vi "Main.vi"() -> ()   [LabVIEW 2023]
doc: "This template is for the Queued Message Handler design pattern.\n\nThe Event Handling Loop generates messages based on user interface actions.\n\nThe Message Handling Loop processes messages generated by the Event Handling Loop, or by other messages. The messages are string values, so new messages can be added easily to the Message Cases case structure in the Message Handling Loop. Each message cluster can also provide an optional value for Message Data, which is a variant that can be converted to whatever message-specific data is required."
uses:
  controls/UI Data.ctl
  support/Message Queue/Enqueue Message (Single).vi
  <vilib>/Utility/file.llb/Write Delimited Spreadsheet (string).vi
  <vilib>/Utility/file.llb/Write Delimited Spreadsheet (DBL).vi
  <vilib>/Instr/_visa.llb/VISA Configure Serial Port (Instr).vi
  <vilib>/Utility/error.llb/Error Cluster From Error Code.vi
  <vilib>/ErrorRing/Error Ring.xnode
  support/Message Queue/Message Queue.lvlib
  support/User Event - Stop/User Event - Stop.lvlib
panel:
  out "Acquiring Read":string
  in  "Step Time (ms)":dbl
  in  "Next Button":bool
  in  "Previous Button":bool
  in  "Test Case":string(combo)="standard"
  in  "File Path":path
  in  "Test Name":string
  out "Torque vs Displacement":cluster{dbl[], dbl[]}(graph)
  in  "COM Port":refnum<visa-resource-name>
  in  "Cycles":dbl
  in  "Torque":dbl
  in  "Microsteps":dbl
  in  "RPM":dbl
  in  "Clear":bool
  in  "Save":bool
  out "Status":string
  in  "Stop":bool
  in  "Start":bool
  in  "Exit":bool
  # "Settings"
  # "Test Controls"
  # "Manual Control"
  # "Torque vs Displacement"
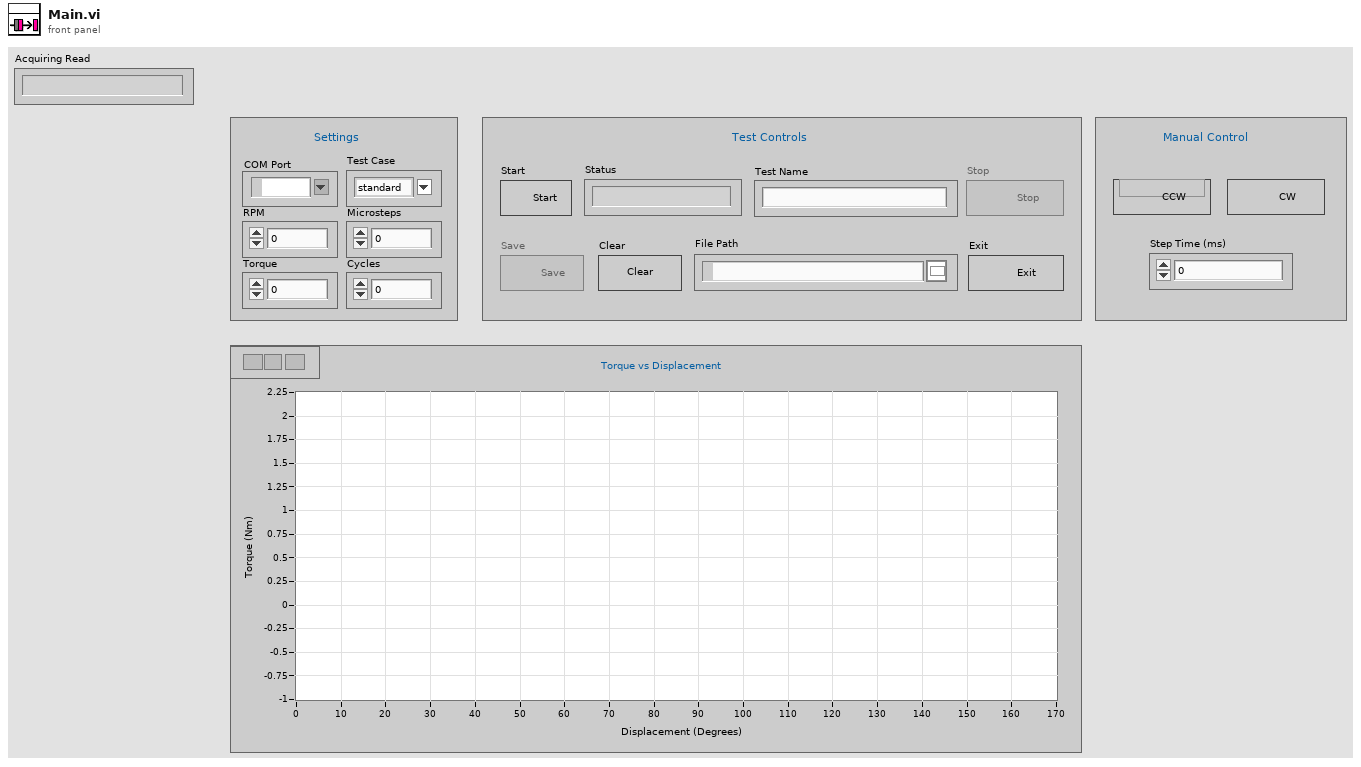
[diagram p1: front panel]
types:
  T1 = cluster{"RPM":dbl, "Microsteps":dbl, "Torque":dbl, "Cycles":dbl, "VISA resource name":refnum<visa-resource-name>, "test case":string}
  T2 = typedef "UI Data.ctl" = cluster{"Start ref":refnum<vi>, "Stop ref":refnum<vi>, "Status ref":refnum<vi>, "Exit ref":refnum<vi>, "Save ref":refnum<vi>, "Clear ref":refnum<vi>, "CCW":refnum<vi>, "CW":refnum<vi>}
  T3 = typedef "Message Queue.lvlib/All Message Queues.ctl" = cluster{"UI":refnum<queue>, "Acquisition":refnum<queue>}
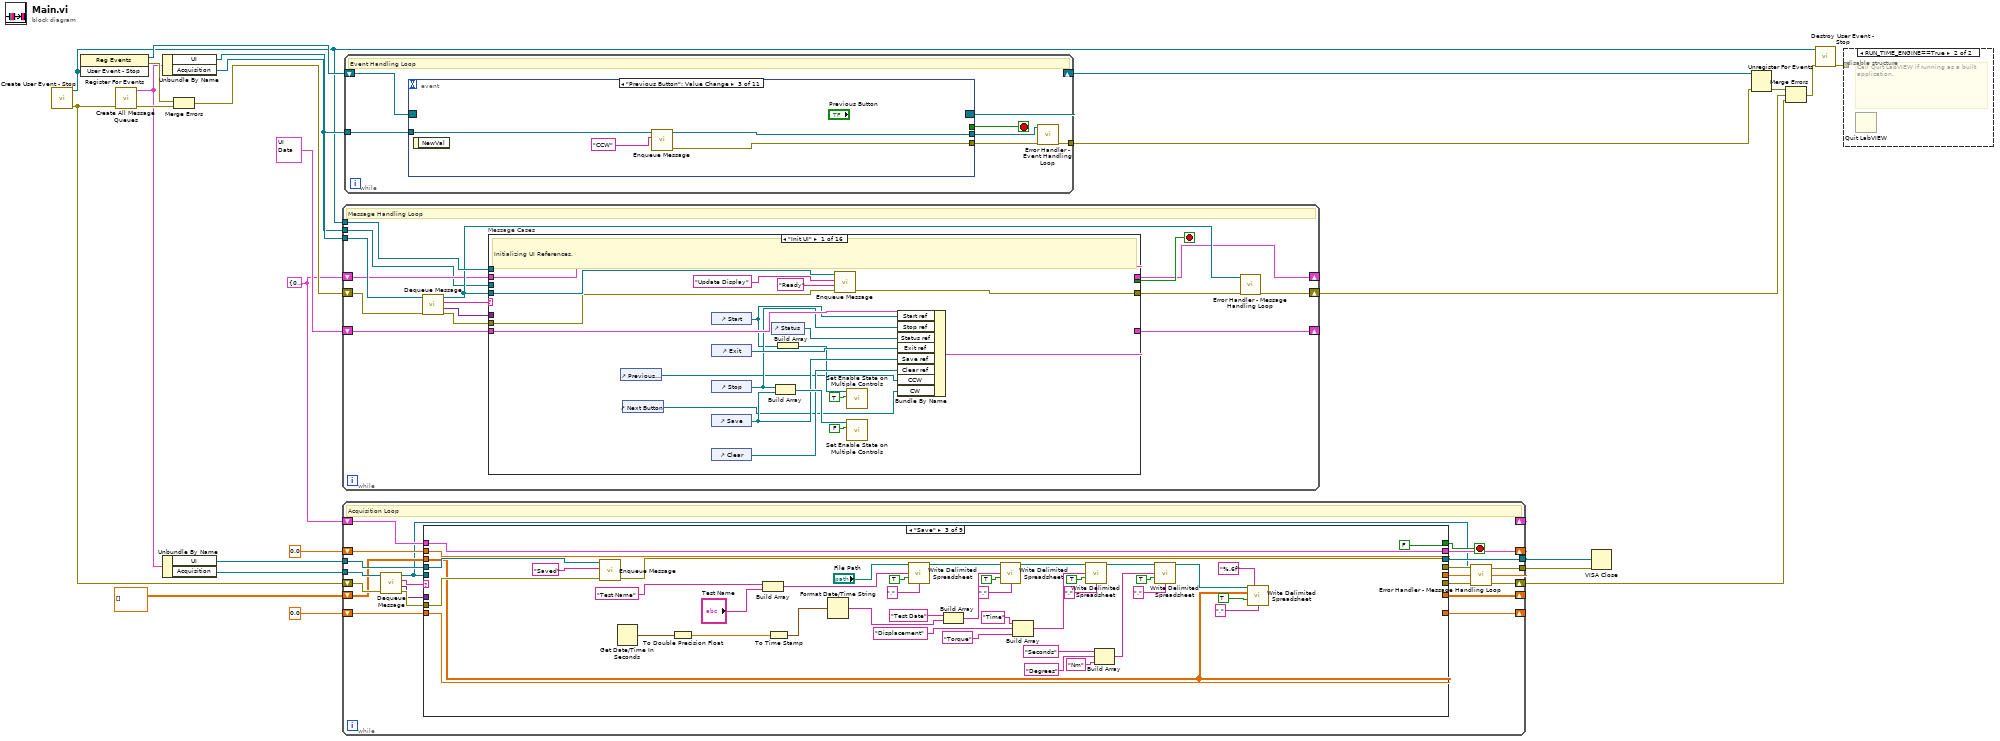
[diagram p0: block diagram]
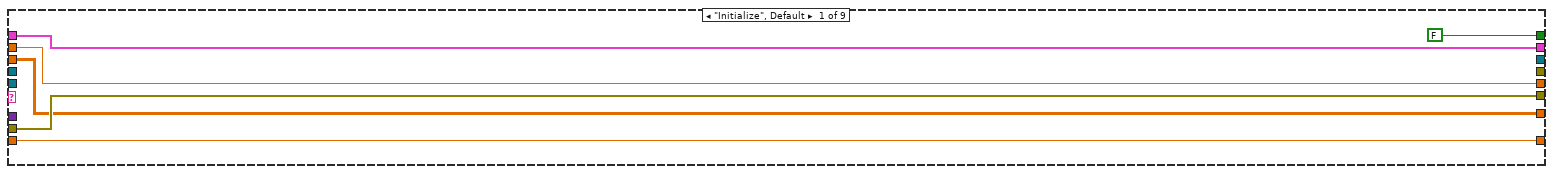
[diagram p2: hidden frame]
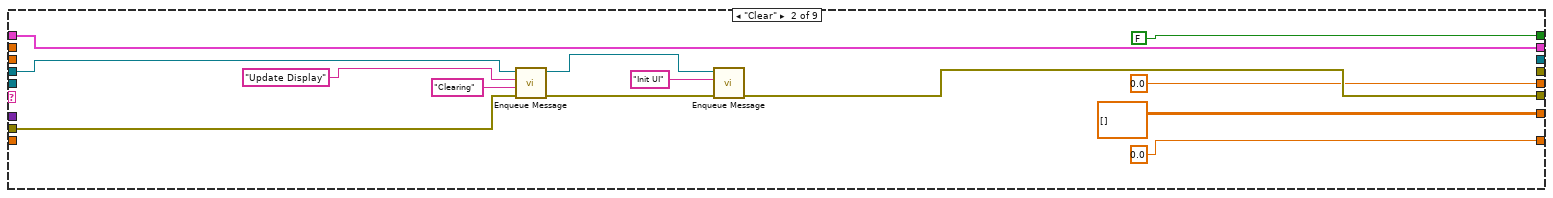
[diagram p3: hidden frame]
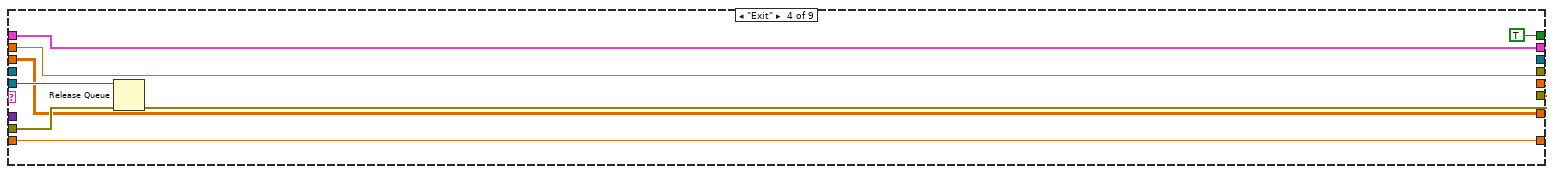
[diagram p4: hidden frame]
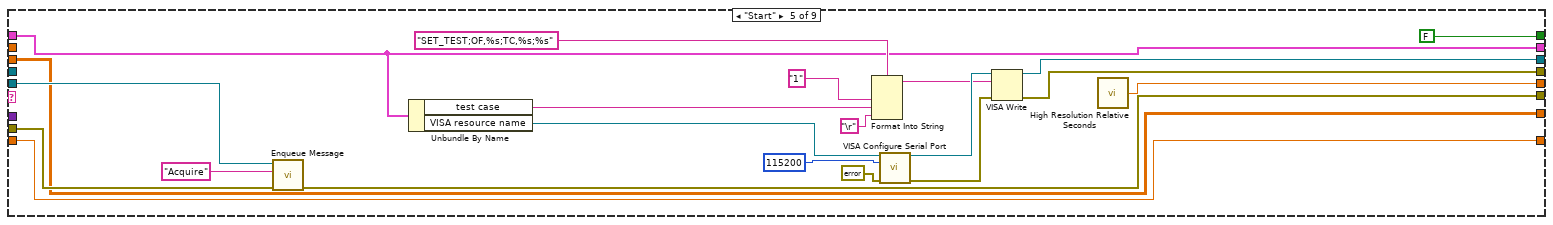
[diagram p5: hidden frame]
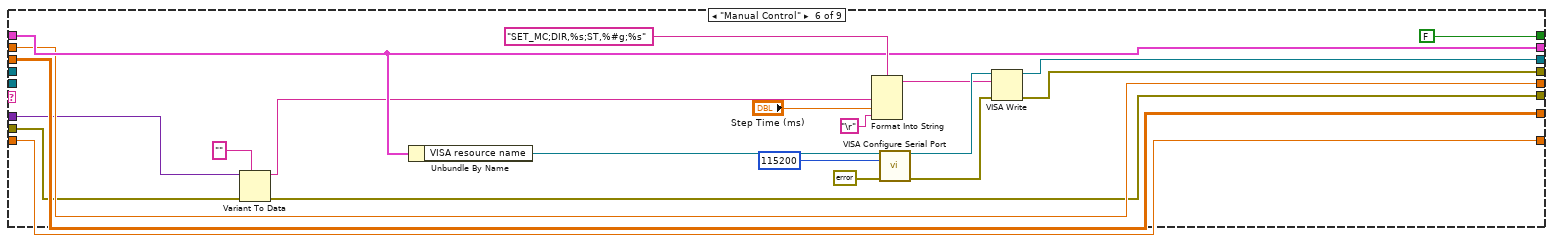
[diagram p6: hidden frame]
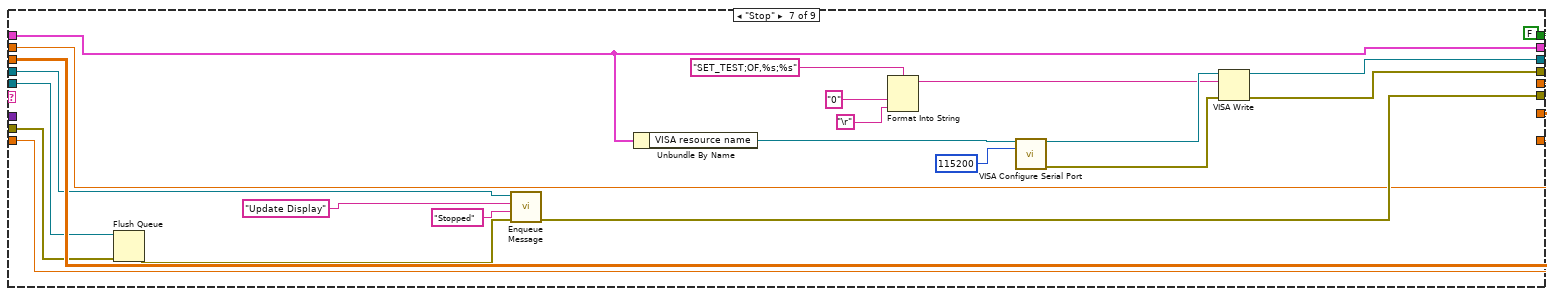
[diagram p7: hidden frame]
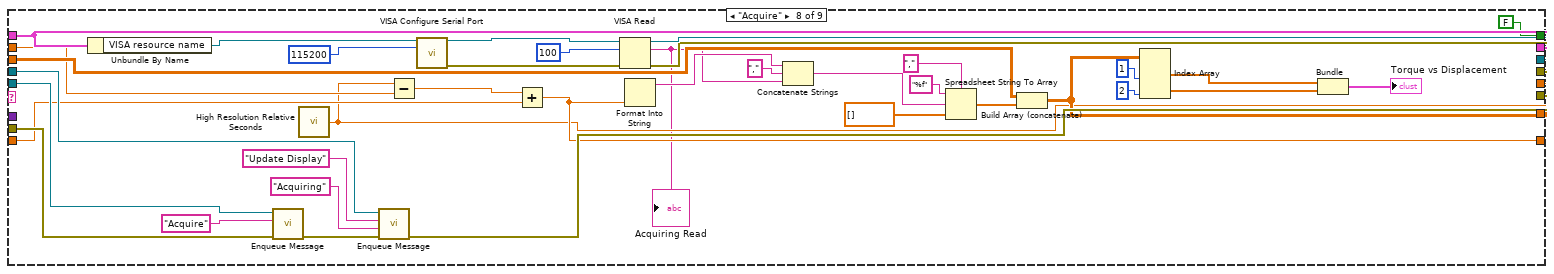
[diagram p8: hidden frame]
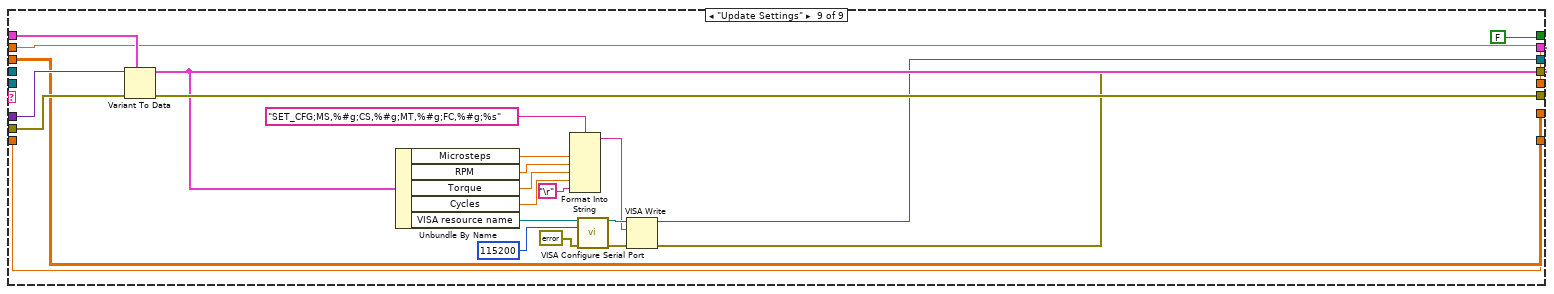
[diagram p9: hidden frame]
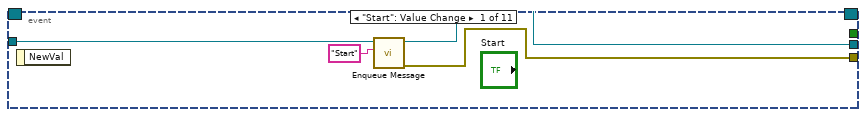
[diagram p11: hidden frame]
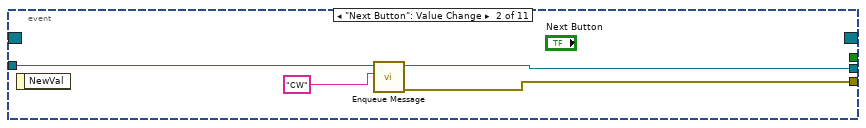
[diagram p12: hidden frame]
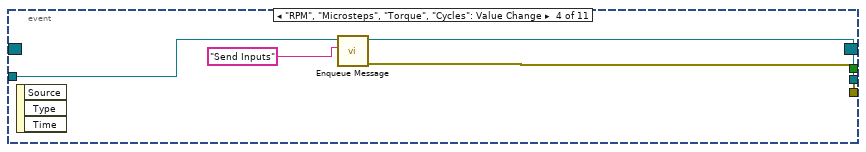
[diagram p13: hidden frame]
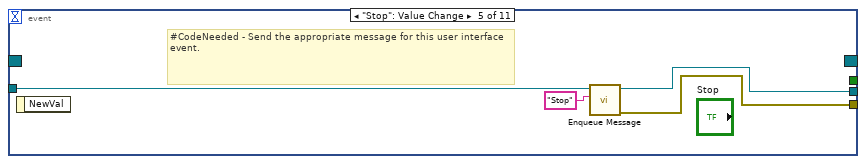
[diagram p14: hidden frame]
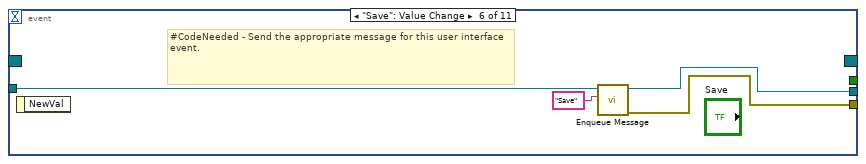
[diagram p15: hidden frame]
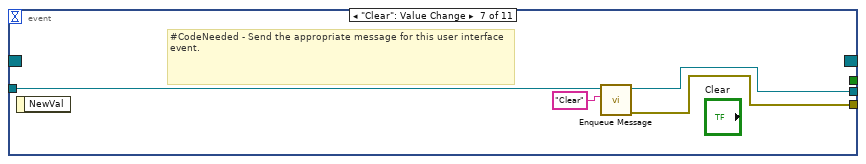
[diagram p16: hidden frame]
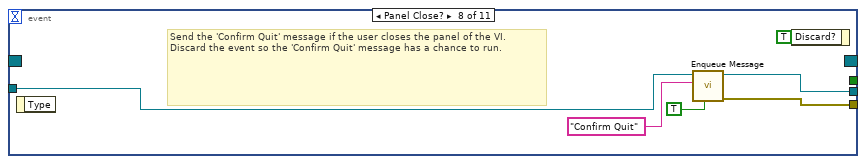
[diagram p17: hidden frame]
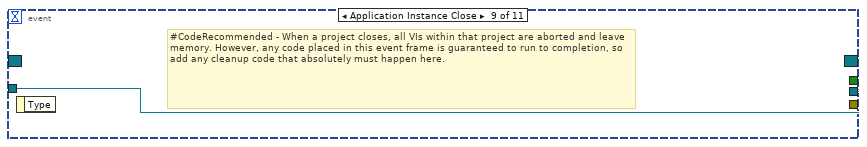
[diagram p18: hidden frame]
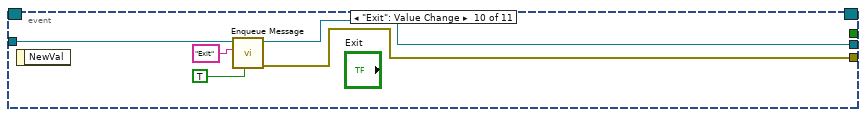
[diagram p19: hidden frame]
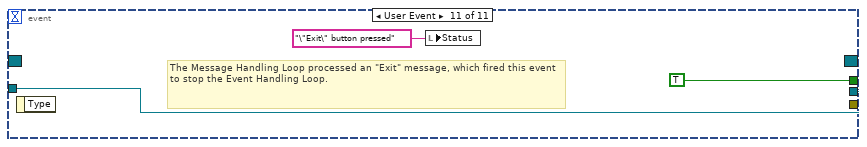
[diagram p20: hidden frame]
diagram:
  w8 = T1 {"RPM"=0.0, "Microsteps"=0.0, "Torque"=0.0, "Cycles"=0.0, "VISA resource name"="", "test case"=""}
  n1 = call "Create User Event - Stop.vi"() -> ("error out"=w9:errorcluster, "User Event - Stop"=w16:refnum<user-event>)  [unwired: 10 in]
  n2 = register-events(w16) -> (reference out=w17:refnum<event-registration>, error out=w14:errorcluster)  [unwired: 2 in]
  n3 = call "Create All Message Queues.vi"("error in (no error)"=w9) -> ("error out"=w25:errorcluster, "Message Queues out"=w11:T3)  [unwired: 9 in]
  n4 = Unbundle By Name(w11) -> ("UI"=w23:refnum<queue>, "Acquisition"=w12:refnum<queue>)
  n5 = Unbundle By Name(w11) -> ("UI"=w7:refnum<queue>, "Acquisition"=w10:refnum<queue>)
  n6 = Merge Errors(w14, w25) -> (w15:errorcluster)
  n7 = while {
    tunnel: w23 -> [w32]
    shift-right: [w39] -> _
    shift-left: T2 {"Start ref"=refnum, "Stop ref"=refnum, "Status ref"=refnum, "Exit ref"=refnum, "Save ref"=refnum, "Clear ref"=refnum, "CCW"=refnum, "CW"=refnum} ("Data Cluster") -> [w40]
    tunnel: w16 -> [w37]
    shift-right: [w28] -> _
    shift-left: w8 -> [w27]
    tunnel: w12 -> [w26]
    shift-right: [w30] -> w24
    shift-left: w15 -> [w36]
    stop <- w38 stop-if-true
    # "Message Handling Loop"
    n8 = call "Dequeue Message.vi"("error in (no error)"=w36, "Message Queue"=w32) -> ("error out"=w35:errorcluster, "Message Data"=w33:variant, "Message"=w34:string, "dup Message Queue"=w31:refnum<queue>)  [unwired: 6 in]
    n9 = case "Message Cases" shown="\"Init UI\"" w34 {
      selector: w34 -> [_ _ _ _ _ _ _ _ _ _ _ _ _ _ _ w208]
      tunnel: w31 -> [w52 w79 w94 _ _ w121 _ _ _ w149 w161 _ _ _ w206 _]
      tunnel: w35 -> [w51 w80 w96 w107 w117 w125 w129 w133 w141 w150 w162 w169 w176 w186 w199 _]
      tunnel: [w60 w81 w101 w108 w111 w123 w127 w136 w144 w159 w165 w172 w179 w193 w202 w209] -> w29
      tunnel: w40 -> [w59 w70 w85 w109 w116 w124 w128 w137 w145 w151 w166 w173 w180 w194 w205 w210]
      tunnel: [w58 w70 w85 w109 w116 w124 w128 w137 w145 w151 w166 w173 w180 w194 w205 w210] -> w39
      tunnel: [_ _ _ _ _ _ _ _ _ _ _ _ _ _ TRUE _] -> w38
      tunnel: w33 -> [_ _ _ w106 w115 _ _ _ _ _ _ _ _ _ _ _]
      tunnel: w37 -> [_ _ _ _ _ _ _ _ _ _ _ _ _ _ w201 _]
      tunnel: w27 -> [w53 w76 w100 w102 w110 w118 w126 w135 w143 w158 w164 w171 w178 w192 w195 w207]
      tunnel: [w53 w76 w100 w102 w110 w118 w126 w135 w143 w158 w164 w171 w178 w185 w195 w207] -> w28
      tunnel: w26 -> [_ w63 w97 _ _ _ _ w132 w140 _ _ w168 w175 w183 w198 _]
      frame "Init UI" {
        # "Initializing UI References."
        n10 = control-ref of="Previous Button"() -> (w42:refnum<vi>)
        n11 = control-ref of="Next Button"() -> (w41:refnum<vi>)
        n12 = control-ref of="Start"() -> (w43:refnum<vi>)
        n13 = control-ref of="Exit"() -> (w56:refnum<vi>)
        n14 = control-ref of="Stop"() -> (w48:refnum<vi>)
        n15 = control-ref of="Save"() -> (w47:refnum<vi>)
        n16 = control-ref of="Clear"() -> (w46:refnum<vi>)
        n17 = control-ref of="Status"() -> (w57:refnum<vi>)
        n18 = Build Array(w48, w47) -> (w49:refnum<vi>[])
        n19 = Build Array(w43) -> (w44:refnum<vi>[])
        n20 = call-poly "Enqueue Message.vi"("error in (no error)"=w51, "Message Data"="Ready" ("Initial Message"), "Message"="Update Display", "Message Queue"=w52) -> ("error out"=w60:errorcluster)  [unwired: 6 in, 1 out]
        n21 = call "Set Enable State on Multiple Controls.vi"("Enable?"=TRUE, "Controls"=w44) -> ()  [unwired: 10 in]
        n22 = call "Set Enable State on Multiple Controls.vi"("Enable?"=FALSE, "Controls"=w49) -> ()  [unwired: 10 in]
        n23 = Bundle By Name(cluster=w59, "Start ref"=w43, "Stop ref"=w48, "Status ref"=w57, "Exit ref"=w56, "Save ref"=w47, "Clear ref"=w46, "CCW"=w42, "CW"=w41) -> (w58:T2)
      }
      frame "Start" {
        # "Starts a test and communicates test start to acquisition loop."
        n24 = Unbundle By Name(w70) -> ("Stop ref"=w67:refnum<vi>, "Start ref"=w65:refnum<vi>, "Exit ref"=w69:refnum<vi>, "Clear ref"=w64:refnum<vi>, "CCW"=w62:refnum<vi>, "CW"=w61:refnum<vi>)
        n25 = Build Array(w65, w69, w64, w62, w61) -> (w71:refnum<vi>[])
        n26 = Build Array(w67) -> (w66:refnum<vi>[])
        n27 = call "Set Enable State on Multiple Controls.vi"("Enable?"=TRUE, "Controls"=w66) -> ()  [unwired: 10 in]
        n28 = call "Set Enable State on Multiple Controls.vi"("Enable?"=FALSE, "Controls"=w71) -> ()  [unwired: 10 in]
        n29 = call-poly "Enqueue Message.vi"("error in (no error)"=w80, "Message Data"="Starting" ("\"Do Something\" button pressed"), "Message"="Update Display", "Message Queue"=w79) -> ("error out"=w75:errorcluster)  [unwired: 6 in, 1 out]
        n30 = call-poly "Enqueue Message.vi"("error in (no error)"=w75, "Message"="Start", "Message Queue"=w63) -> ("error out"=w73:errorcluster)  [unwired: 7 in, 1 out]
        n31 = Merge Errors(w73) -> (w81:errorcluster)
      }
      frame "Stop" {
        # "Something - Replace this message with functionality for your own application."
        n32 = Unbundle By Name(w85) -> ("CCW"=w82:refnum<vi>, "CW"=w83:refnum<vi>, "Save ref"=w90:refnum<vi>, "Exit ref"=w84:refnum<vi>, "Stop ref"=w89:refnum<vi>)
        n33 = Build Array(w82, w83, w90, w84) -> (w91:refnum<vi>[])
        n34 = Build Array(w89) -> (w88:refnum<vi>[])
        n35 = call "Set Enable State on Multiple Controls.vi"("Enable?"=TRUE, "Controls"=w91) -> ()  [unwired: 10 in]
        n36 = call "Set Enable State on Multiple Controls.vi"("Enable?"=FALSE, "Controls"=w88) -> ()  [unwired: 10 in]
        n37 = call-poly "Enqueue Message.vi"("error in (no error)"=w96, "Message Data"="Stopping" ("Message"), "Message"="Update Display", "Message Queue"=w94) -> ("error out"=w95:errorcluster)  [unwired: 6 in, 1 out]
        n38 = call-poly "Enqueue Message.vi"("error in (no error)"=w95, "Message"="Stop", "Message Queue"=w97) -> ("error out"=w99:errorcluster)  [unwired: 7 in, 1 out]
        n39 = Merge Errors(w99) -> (w101:errorcluster)
      }
      frame "Update Display" {
        # "Update Display - Convert the message data to a string to display in the Data Display indicator."
        n40 = Variant To Data(error in=w107, type="", Variant=w106) -> (data=→"Status":string, error out=w104:errorcluster)
        n41 = Merge Errors(w104) -> (w108:errorcluster)
      }
      frame "Error" {
        # "Error - Display an error dialog. This message is sent by the \"Error Handler\" VIs at the end of other loops in this application."
        n42 = Variant To Data(error in=w117, type=errorcluster {"status"=FALSE, "code"=0, "source"=""} ("error constant"), Variant=w115) -> (data=w113:errorcluster, error out=w112:errorcluster)
        n43 = call <vilib>:"Simple Error Handler.vi"("error in (no error)"=w113) -> ()  [unwired: 4 in, 5 out]
        n44 = Merge Errors(w112) -> (w111:errorcluster)
      }
      frame "Confirm Quit" {
        # "#CodeNeeded - If you want to provide an \"Are you sure\" dialog (or some other notification) before the application exits, place that code here. This message is typically sent from a Panel Close? event."
        # "Confirm Quit - Message that can confirm whether or not the user wants to exit the application."
        n45 = call-poly "Enqueue Message.vi"("Priority Message? (F)"=TRUE, "error in (no error)"=w125, "Message"="Exit", "Message Queue"=w121) -> ("error out"=w122:errorcluster)  [unwired: 6 in, 1 out]
        n46 = Merge Errors(w122) -> (w123:errorcluster)
      }
      frame "---Copy This Frame---" {
        # "Duplicate this frame when creating new messages.  Change this comment in the duplicated frame to describe this message."
        n47 = Merge Errors(w129) -> (w127:errorcluster)
      }
      frame "CW" {
        # "Duplicate this frame when creating new messages.  Change this comment in the duplicated frame to describe this message."
        n48 = call-poly "Enqueue Message.vi"("error in (no error)"=w133, "Message Data"="CW", "Message"="Manual Control", "Message Queue"=w132) -> ("error out"=w134:errorcluster)  [unwired: 6 in, 1 out]
        n49 = Merge Errors(w134) -> (w136:errorcluster)
      }
      frame "CCW" {
        # "Duplicate this frame when creating new messages.  Change this comment in the duplicated frame to describe this message."
        n50 = call-poly "Enqueue Message.vi"("error in (no error)"=w141, "Message Data"="CCW", "Message"="Manual Control", "Message Queue"=w140) -> ("error out"=w142:errorcluster)  [unwired: 6 in, 1 out]
        n51 = Merge Errors(w142) -> (w144:errorcluster)
      }
      frame "Saved" {
        # "Duplicate this frame when creating new messages.  Change this comment in the duplicated frame to describe this message."
        n52 = Unbundle By Name(w151) -> ("Clear ref"=w157:refnum<vi>, "Save ref"=w155:refnum<vi>)
        n53 = Build Array(w155) -> (w156:refnum<vi>[])
        n54 = Build Array(w157) -> (w154:refnum<vi>[])
        n55 = call "Set Enable State on Multiple Controls.vi"("Enable?"=FALSE, "Controls"=w156) -> ()  [unwired: 10 in]
        n56 = call "Set Enable State on Multiple Controls.vi"("Enable?"=TRUE, "Controls"=w154) -> ()  [unwired: 10 in]
        n57 = call-poly "Enqueue Message.vi"("error in (no error)"=w150, "Message Data"="Saved" ("Message"), "Message"="Update Display", "Message Queue"=w149) -> ("error out"=w146:errorcluster)  [unwired: 6 in, 1 out]
        n58 = Merge Errors(w146) -> (w159:errorcluster)
      }
      frame "Initialize" {
        # "Duplicate this frame when creating new messages.  Change this comment in the duplicated frame to describe this message."
        n59 = call-poly "Enqueue Message.vi"("error in (no error)"=w162, "Message"="Init UI", "Message Queue"=w161) -> ("error out"=w163:errorcluster)  [unwired: 7 in, 1 out]
        n60 = Merge Errors(w163) -> (w165:errorcluster)
      }
      frame "Clear" {
        # "Sends clear message to acquisition loop to clear recorded data."
        n61 = call-poly "Enqueue Message.vi"("error in (no error)"=w169, "Message"="Clear", "Message Queue"=w168) -> ("error out"=w170:errorcluster)  [unwired: 7 in, 1 out]
        n62 = Merge Errors(w170) -> (w172:errorcluster)
      }
      frame "Save" {
        # "Saves Current Data"
        n63 = call-poly "Enqueue Message.vi"("error in (no error)"=w176, "Message"="Save", "Message Queue"=w175) -> ("error out"=w177:errorcluster)  [unwired: 7 in, 1 out]
        n64 = Merge Errors(w177) -> (w179:errorcluster)
      }
      frame "Send Inputs" {
        # "Send updated inputs to acquistion loop."
        n65 = Bundle By Name(cluster=w192, "RPM"="RPM", "Microsteps"="Microsteps", "Torque"="Torque", "Cycles"="Cycles", "VISA resource name"="COM Port", "test case"="Test Case") -> (w185:T1)
        n66 = call-poly "Enqueue Message.vi"("error in (no error)"=w186, "Message Data"=w185, "Message"="Update Settings", "Message Queue"=w183) -> ("error out"=w181:errorcluster)  [unwired: 6 in, 1 out]
        n67 = Merge Errors(w181) -> (w193:errorcluster)
      }
      frame "Exit" {
        # "Stop the VI"
        # "Release the message queue reference"
        # "Exit - Exit the application."
        n68 = Release Queue(queue=w206, error in (no error)=w199) -> (error out=w203:errorcluster)  [unwired: 1 in, 2 out]
        n69 = call-poly "Enqueue Message.vi"("Priority Message? (F)"=TRUE, "Message"="Exit", "Message Queue"=w198) -> ()  [unwired: 7 in, 2 out]
        n70 = call "Fire User Event - Stop.vi"("User Event - Stop"=w201) -> ("error out"=w200:errorcluster)  [unwired: 10 in]
        n71 = Merge Errors(w200, w203) -> (w202:errorcluster)
      }
      frame Default {
        # "'Default' case only runs if there is a message that isn't defined in any of the other cases.  Output a programming error."
        n72 = xnode "Error Ring"("parameter 0"=w208) -> ("error out"=w209:errorcluster)
      }
    }
    n73 = call "Error Handler - Message Handling Loop.vi"("error in (no error)"=w29, "Message Queue"=w31) -> ("dup error in"=w30:errorcluster)  [unwired: 8 in, 1 out]
  }
  n74 = while {
    tunnel: w10 -> [w237]
    shift-right: [w219] -> w6
    shift-left: w9 -> [w236]
    shift-right: [w231] -> _
    shift-left: w8 -> [w234]
    tunnel: w7 -> [w227]
    tunnel: [w229] -> w5
    tunnel: [w228] -> w4
    shift-right: [w225] -> _
    shift-left: dbl[][] [] -> [w226]
    shift-right: [w224] -> _
    shift-left: 0.0 -> [w223]
    shift-right: [w222] -> _
    shift-left: 0.0 -> [w221]
    stop <- w230 stop-if-true
    # "Acquisition Loop"
    n75 = call "Dequeue Message.vi"("error in (no error)"=w236, "Message Queue"=w237) -> ("error out"=w235:errorcluster, "Message Data"=w232:variant, "Message"=w233:string, "dup Message Queue"=w218:refnum<queue>)  [unwired: 6 in]
    n76 = case shown="\"Save\"" w233 {
      tunnel: w235 -> [w241 w254 w295 w303 w316 w331 w357 w399 w428]
      tunnel: w234 -> [w243 w256 w298 w306 w319 w342 w362 w405 w429]
      tunnel: w232 -> [_ _ _ _ _ w329 _ _ w430]
      tunnel: [w243 w256 w298 w306 w319 w342 w362 w405 w416] -> w231
      tunnel: [FALSE FALSE FALSE TRUE FALSE FALSE FALSE FALSE FALSE] -> w230
      tunnel: w218 -> [_ _ _ w304 w313 _ w358 w400 _]
      tunnel: [_ _ _ _ w317 w341 w361 w402 w409] -> w229
      tunnel: [_ _ _ _ w315 w340 w360 w401 w408] -> w228
      tunnel: w227 -> [_ w253 w296 _ _ _ w354 w395 _]
      tunnel: [w241 w248 w257 w302 w312 w330 w355 w396 w427] -> w220
      tunnel: w226 -> [w240 _ w290 w301 w311 w338 w359 w388 w426]
      tunnel: [w240 dbl[][] [] w290 w301 w311 w338 w359 w378 w426] -> w225
      tunnel: [w239 0.0 w271 w300 w310 w337 w352 w374 w425] -> w224
      tunnel: w223 -> [w239 _ w271 w300 w310 w337 w352 w377 w425]
      tunnel: [w238 0.0 w268 w299 w309 w335 w351 w373 w424] -> w222
      tunnel: w221 -> [w238 _ w268 w299 _ w335 w351 w376 w424]
      frame "Initialize", Default {
      }
      frame "Clear" {
        n77 = call-poly "Enqueue Message.vi"("error in (no error)"=w254, "Message Data"="Clearing" ("Message"), "Message"="Update Display", "Message Queue"=w253) -> ("error out"=w249:errorcluster, "dup Message Queue"=w250:refnum<queue>)  [unwired: 6 in]
        n78 = call-poly "Enqueue Message.vi"("error in (no error)"=w249, "Message"="Init UI", "Message Queue"=w250) -> ("error out"=w248:errorcluster)  [unwired: 7 in, 1 out]
      }
      frame "Save" {
        n79 = call-poly "Enqueue Message.vi"("error in (no error)"=w295, "Message"="Saved", "Message Queue"=w296) -> ("error out"=w257:errorcluster)  [unwired: 7 in, 1 out]
        n80 = Get Date/Time In Seconds() -> (seconds since 1Jan1904=w266:timestamp)
        n81 = To Double Precision Float(number=w266) -> (double precision float=w267:dbl)
        n82 = Build Array("Test Name" ("delimiter (\\t)"), "Test Name") -> (w288:string[])
        n83 = To Time Stamp(1:w267) -> (0:w263:timestamp)
        n84 = Format Date/Time String(seconds (now)=w263) -> (date/time string=w259:string)  [unwired: 2 in]
        n85 = call-poly <vilib>:"Write Delimited Spreadsheet.vi"("file path (dialog if empty)"="File Path", "1D data"=w288, "append to file? (new file:F)"=TRUE, "delimiter (\\t)"="," ("delimiter (\\t)")) -> ("new file path (Not A Path if cancelled)"=w262:path)  [unwired: 10 in, 1 out]
        n86 = Build Array("Test Date" ("delimiter (\\t)"), w259) -> (w258:string[])
        n87 = call-poly <vilib>:"Write Delimited Spreadsheet.vi"("file path (dialog if empty)"=w262, "1D data"=w258, "append to file? (new file:F)"=TRUE, "delimiter (\\t)"="," ("delimiter (\\t)")) -> ("new file path (Not A Path if cancelled)"=w261:path)  [unwired: 10 in, 1 out]
        n88 = Build Array("Time" ("element"), "Displacement" ("delimiter (\\t)"), "Torque" ("delimiter (\\t)")) -> (w282:string[])
        n89 = call-poly <vilib>:"Write Delimited Spreadsheet.vi"("file path (dialog if empty)"=w261, "1D data"=w282, "append to file? (new file:F)"=TRUE, "delimiter (\\t)"="," ("delimiter (\\t)")) -> ("new file path (Not A Path if cancelled)"=w280:path)  [unwired: 10 in, 1 out]
        n90 = Build Array("Seconds" ("element"), "Degrees" ("delimiter (\\t)"), "Nm" ("delimiter (\\t)")) -> (w281:string[])
        n91 = call-poly <vilib>:"Write Delimited Spreadsheet.vi"("file path (dialog if empty)"=w280, "1D data"=w281, "append to file? (new file:F)"=TRUE, "delimiter (\\t)"="," ("delimiter (\\t)")) -> ("new file path (Not A Path if cancelled)"=w279:path)  [unwired: 10 in, 1 out]
        n92 = call-poly <vilib>:"Write Delimited Spreadsheet.vi"("file path (dialog if empty)"=w279, "format (%.3f)"="%.6f", "2D data"=w290, "append to file? (new file:F)"=TRUE, "delimiter (\\t)"="," ("delimiter (\\t)")) -> ()  [unwired: 9 in, 2 out]
      }
      frame "Exit" {
        n93 = Release Queue(queue=w304, error in (no error)=w303) -> (error out=w302:errorcluster)  [unwired: 1 in, 2 out]
      }
      frame "Start" {
        n94 = call-poly "Enqueue Message.vi"("error in (no error)"=w316, "Message"="Acquire", "Message Queue"=w313) -> ("error out"=w312:errorcluster)  [unwired: 7 in, 1 out]
        n95 = Unbundle By Name(w319) -> ("test case"=w307:string, "VISA resource name"=w324:refnum<visa-resource-name>)
        n96 = Format Into String(format string="SET_TEST;OF,%s;TC,%s;%s", "1", w307, "\r") -> (resulting string=w320:string)  [unwired: 2 in, 1 out]
        n97 = call-poly "VISA Configure Serial Port"("VISA resource name"=w324, "baud rate (9600)"=u32 115200, "error in (no error)"=errorcluster {"status"=FALSE, "code"=0, "source"=""}) -> ("VISA resource name out"=w321:refnum<visa-resource-name>, "error out"=w322:errorcluster)  [unwired: 11 in]
        n98 = VISA Write(VISA resource name=w321, write buffer=w320, error in (no error)=w322) -> (VISA resource name out=w317:refnum<visa-resource-name>, error out=w315:errorcluster)  [unwired: 1 out]
        n99 = call <vilib>:"High Resolution Relative Seconds.vi"() -> ("relative seconds"=w309:dbl)
      }
      frame "Manual Control" {
        n100 = Variant To Data(error in=w331, type="", Variant=w329) -> (data=w328:string, error out=w330:errorcluster)
        n101 = Unbundle By Name(w342) -> ("VISA resource name"=w347:refnum<visa-resource-name>)
        n102 = Format Into String(format string="SET_MC;DIR,%s;ST,%#g;%s", w328, "Step Time (ms)", "\r") -> (resulting string=w343:string)  [unwired: 2 in, 1 out]
        n103 = call-poly "VISA Configure Serial Port"("VISA resource name"=w347, "baud rate (9600)"=u32 115200, "error in (no error)"=errorcluster {"status"=FALSE, "code"=0, "source"=""}) -> ("VISA resource name out"=w344:refnum<visa-resource-name>, "error out"=w345:errorcluster)  [unwired: 11 in]
        n104 = VISA Write(VISA resource name=w344, write buffer=w343, error in (no error)=w345) -> (VISA resource name out=w341:refnum<visa-resource-name>, error out=w340:errorcluster)  [unwired: 1 out]
      }
      frame "Stop" {
        n105 = Flush Queue(queue=w358, error in (no error)=w357) -> (error out=w356:errorcluster)  [unwired: 2 out]
        n106 = call-poly "Enqueue Message.vi"("error in (no error)"=w356, "Message Data"="Stopped" ("Message"), "Message"="Update Display", "Message Queue"=w354) -> ("error out"=w355:errorcluster)  [unwired: 6 in, 1 out]
        n107 = Unbundle By Name(w362) -> ("VISA resource name"=w367:refnum<visa-resource-name>)
        n108 = Format Into String(format string="SET_TEST;OF,%s;%s", "0", "\r") -> (resulting string=w363:string)  [unwired: 2 in, 1 out]
        n109 = call-poly "VISA Configure Serial Port"("VISA resource name"=w367, "baud rate (9600)"=u32 115200) -> ("VISA resource name out"=w364:refnum<visa-resource-name>, "error out"=w365:errorcluster)  [unwired: 12 in]
        n110 = VISA Write(VISA resource name=w364, write buffer=w363, error in (no error)=w365) -> (VISA resource name out=w361:refnum<visa-resource-name>, error out=w360:errorcluster)  [unwired: 1 out]
      }
      frame "Acquire" {
        n111 = Unbundle By Name(w405) -> ("VISA resource name"=w407:refnum<visa-resource-name>)
        n112 = call-poly "Enqueue Message.vi"("error in (no error)"=w399, "Message"="Acquire", "Message Queue"=w400) -> ("error out"=w397:errorcluster)  [unwired: 7 in, 1 out]
        n113 = call <vilib>:"High Resolution Relative Seconds.vi"() -> ("relative seconds"=w373:dbl)
        n114 = call-poly "Enqueue Message.vi"("error in (no error)"=w397, "Message Data"="Acquiring" ("\"Do Something\" button pressed"), "Message"="Update Display", "Message Queue"=w395) -> ("error out"=w396:errorcluster)  [unwired: 6 in, 1 out]
        n115 = Subtract(x=w373, y=w376) -> (x-y=w375:dbl)
        n116 = call-poly "VISA Configure Serial Port"("VISA resource name"=w407, "baud rate (9600)"=u32 115200) -> ("VISA resource name out"=w404:refnum<visa-resource-name>, "error out"=w403:errorcluster)  [unwired: 12 in]
        n117 = Add(x=w375, y=w377) -> (x+y=w374:dbl)
        n118 = VISA Read(VISA resource name=w404, byte count=u32 100, error in (no error)=w403) -> (VISA resource name out=w402:refnum<visa-resource-name>, read buffer=w371:string, error out=w401:errorcluster)  [unwired: 1 out]
        "Acquiring Read" <- w371
        n119 = Format Into String(w374) -> (resulting string=w379:string)  [unwired: 3 in, 1 out]
        n120 = Concatenate Strings(w379, "," ("string"), w371) -> (w380:string)
        n121 = Spreadsheet String To Array(delimiter (Tab)=",", format string="%f", spreadsheet string=w380, array type (2D Dbl)=dbl[] []) -> (array=w387:dbl[])
        n122 = Build Array (concatenate)(w388, w387) -> (w378:dbl[][])
        n123 = Index Array(array=w378, index (col) #1=1 ("index (col)"), index (col) #2=2 ("index (col)")) -> (element #1=w384:dbl[], element #2=w383:dbl[])  [unwired: 2 in]
        n124 = Bundle(w384, w383) -> (→"Torque vs Displacement":cluster{dbl[], dbl[]})  [unwired: 1 in]
      }
      frame "Update Settings" {
        n125 = Variant To Data(error in=w428, type=w429, Variant=w430) -> (data=w416:T1, error out=w427:errorcluster)
        n126 = Unbundle By Name(w416) -> ("Microsteps"=w415:dbl, "RPM"=w410:dbl, "Torque"=w411:dbl, "Cycles"=w412:dbl, "VISA resource name"=w413:refnum<visa-resource-name>)
        n127 = Format Into String(format string="SET_CFG;MS,%#g;CS,%#g;MT,%#g;FC,%#g;%s", w415, w410, w411, w412, "\r") -> (resulting string=w419:string)  [unwired: 2 in, 1 out]
        n128 = call-poly "VISA Configure Serial Port"("VISA resource name"=w413, "baud rate (9600)"=u32 115200, "error in (no error)"=errorcluster {"status"=FALSE, "code"=0, "source"=""}) -> ("VISA resource name out"=w420:refnum<visa-resource-name>, "error out"=w418:errorcluster)  [unwired: 11 in]
        n129 = VISA Write(VISA resource name=w420, write buffer=w419, error in (no error)=w418) -> (VISA resource name out=w409:refnum<visa-resource-name>, error out=w408:errorcluster)  [unwired: 1 out]
      }
    }
    n130 = call "Error Handler - Message Handling Loop.vi"("error in (no error)"=w220, "Message Queue"=w218) -> ("dup error in"=w219:errorcluster)  [unwired: 8 in, 1 out]
  }
  n131 = while {
    tunnel: w23 -> [w437]
    shift-right: [w435] -> w20
    shift-left: w17 -> [w436]
    tunnel: [w431] -> w18
    stop <- w433 stop-if-true
    # "Event Handling Loop"
    n132 = event shown="[2] \"Previous Button\": Value Change" {
      selector: w436 -> [_ _ _ _ _ _ _ _ _ _ _]
      dyn-events: [_ _ _ _ _ _ _ _ _ _ _] -> w435
      timeout: _ -> [_ _ _ _ _ _ _ _ _ _ _]
      tunnel: [_ _ _ _ _ _ _ _ _ _ TRUE ("Discard?")] -> w433
      tunnel: w437 -> [w441 w445 w449 w453 w457 w461 w465 w470 w472 w477 w480]
      tunnel: [w438 w442 w446 w450 w454 w458 w462 w469 _ w476 _] -> w434
      tunnel: [w440 w444 w448 w452 w456 w460 w464 w468 w472 w475 w480] -> w432
      event "Start": Value Change {
        n133 = event-data() -> ()  [unwired: 1 in, 1 out]
        n134 = call-poly "Enqueue Message.vi"("Message"="Start", "Message Queue"=w441) -> ("error out"=w438:errorcluster, "dup Message Queue"=w440:refnum<queue>)  [unwired: 8 in]
      }
      event "Next Button": Value Change {
        n135 = event-data() -> ()  [unwired: 1 in, 1 out]
        n136 = call-poly "Enqueue Message.vi"("Message"="CW", "Message Queue"=w445) -> ("error out"=w442:errorcluster, "dup Message Queue"=w444:refnum<queue>)  [unwired: 8 in]
      }
      event "Previous Button": Value Change {
        n137 = event-data() -> ()  [unwired: 1 in, 1 out]
        n138 = call-poly "Enqueue Message.vi"("Message"="CCW", "Message Queue"=w449) -> ("error out"=w446:errorcluster, "dup Message Queue"=w448:refnum<queue>)  [unwired: 8 in]
      }
      event "RPM", "Microsteps", "Torque", "Cycles": Value Change {
        n139 = event-data() -> ()  [unwired: 1 in, 3 out]
        n140 = call-poly "Enqueue Message.vi"("Message"="Send Inputs", "Message Queue"=w453) -> ("error out"=w450:errorcluster, "dup Message Queue"=w452:refnum<queue>)  [unwired: 8 in]
      }
      event "Stop": Value Change {
        # "#CodeNeeded - Send the appropriate message for this user interface event."
        n141 = event-data() -> ()  [unwired: 1 in, 1 out]
        n142 = call-poly "Enqueue Message.vi"("Message"="Stop", "Message Queue"=w457) -> ("error out"=w454:errorcluster, "dup Message Queue"=w456:refnum<queue>)  [unwired: 8 in]
      }
      event "Save": Value Change {
        # "#CodeNeeded - Send the appropriate message for this user interface event."
        n143 = event-data() -> ()  [unwired: 1 in, 1 out]
        n144 = call-poly "Enqueue Message.vi"("Message"="Save", "Message Queue"=w461) -> ("error out"=w458:errorcluster, "dup Message Queue"=w460:refnum<queue>)  [unwired: 8 in]
      }
      event "Clear": Value Change {
        # "#CodeNeeded - Send the appropriate message for this user interface event."
        n145 = event-data() -> ()  [unwired: 1 in, 1 out]
        n146 = call-poly "Enqueue Message.vi"("Message"="Clear", "Message Queue"=w465) -> ("error out"=w462:errorcluster, "dup Message Queue"=w464:refnum<queue>)  [unwired: 8 in]
      }
      event Panel Close? {
        # "Send the 'Confirm Quit' message if the user closes the panel of the VI. Discard the event so the 'Confirm Quit' message has a chance to run."
        n147 = event-data() -> ()  [unwired: 1 in, 1 out]
        n148 = call-poly "Enqueue Message.vi"("Priority Message? (F)"=TRUE, "Message"="Confirm Quit", "Message Queue"=w470) -> ("error out"=w469:errorcluster, "dup Message Queue"=w468:refnum<queue>)  [unwired: 7 in]
        n149 = event-data("Discard?"=TRUE) -> ()  [unwired: 1 in, 1 out]
      }
      event Application Instance Close {
        # "#CodeRecommended - When a project closes, all VIs within that project are aborted and leave memory. However, any code placed in this event frame is guaranteed to run to completion, so add any cleanup code that absolutely must happen here."
        n150 = event-data() -> ()  [unwired: 1 in, 1 out]
      }
      event "Exit": Value Change {
        n151 = event-data() -> ()  [unwired: 1 in, 1 out]
        n152 = call-poly "Enqueue Message.vi"("Priority Message? (F)"=TRUE, "Message"="Exit", "Message Queue"=w477) -> ("error out"=w476:errorcluster, "dup Message Queue"=w475:refnum<queue>)  [unwired: 7 in]
      }
      event User Event {
        # "The Message Handling Loop processed an \"Exit\" message, which fired this event to stop the Event Handling Loop."
        n153 = event-data() -> ()  [unwired: 1 in, 1 out]
        n154 = local write "Status"("\"Exit\" button pressed" ("VI Stopped")) -> ()
      }
    }
    n155 = call "Error Handler - Event Handling Loop.vi"("error in (no error)"=w434, "Message Queue"=w432) -> ("dup error in"=w431:errorcluster)  [unwired: 8 in, 1 out]
  }
  n156 = VISA Close(VISA resource name=w5, error in (no error)=w4) -> ()  [unwired: 1 out]
  n157 = Unregister For Events(event registration refnum=w20, error in=w18) -> (error out=w21:errorcluster)
  n158 = Merge Errors(w21, w24, w6) -> (w22:errorcluster)
  n159 = call "Destroy User Event - Stop.vi"("error in (no error)"=w22, "User Event - Stop"=w16) -> ("error out"=w19:errorcluster)  [unwired: 9 in]
  n160 = disable-structure shown="RUN_TIME_ENGINE==True" {
    disable-tunnel: w19 -> [_ _]
    frame condition #0 (active) {
    }
    frame condition #1 {
      # "Call Quit LabVIEW if running as a built application."
      n161 = Quit LabVIEW() -> ()  [unwired: 1 in]
    }
  }
